vi "maxigauge_get_p.vi"(8 "err_in":errorcluster, 10 "sensor_number":i32=1, 11 "visa_in":refnum<visa-resource-name>="COM8") -> (0 "err_out":errorcluster, 2 "pressure":dbl caption="Torr", 3 "visa_out":refnum<visa-resource-name>, 4 "status":bool)   [LabVIEW 2019]
panel:
  out "read_2":string
  out "read_1":string
  out "status_ack":bool
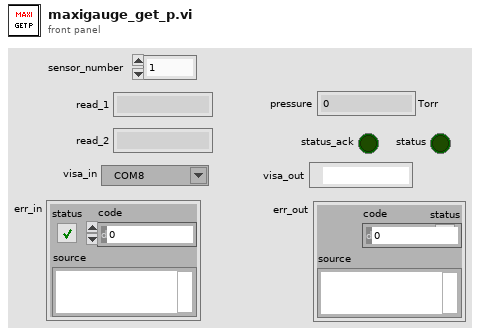
[diagram p1: front panel]
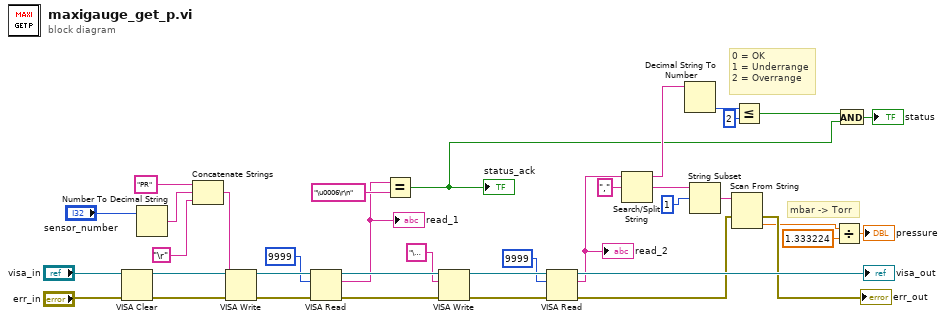
[diagram p0: block diagram]
diagram:
  # "0 = OK\n1 = Underrange\n2 = Overrange"
  # "mbar -> Torr"
  n1 = VISA Clear(VISA resource name="visa_in", error in (no error)="err_in") -> (VISA resource name out=w13:refnum<visa-resource-name>, error out=w11:errorcluster)
  n2 = Number To Decimal String(number="sensor_number") -> (decimal integer string=w16:string)  [unwired: 1 in]
  n3 = Concatenate Strings("PR" ("string"), w16, "\r") -> (w17:string)
  n4 = VISA Write(VISA resource name=w13, write buffer=w17, error in (no error)=w11) -> (VISA resource name out=w36:refnum<visa-resource-name>, error out=w37:errorcluster)  [unwired: 1 out]
  n5 = VISA Read(VISA resource name=w36, byte count=u32 9999, error in (no error)=w37) -> (VISA resource name out=w34:refnum<visa-resource-name>, read buffer=w23:string, error out=w33:errorcluster)  [unwired: 1 out]
  "read_1" <- w23
  n6 = Equal?(x=w23, y="\u0006\r\n") -> (x = y?=w20:bool)
  "status_ack" <- w20
  n7 = VISA Write(VISA resource name=w34, write buffer="\u0005", error in (no error)=w33) -> (VISA resource name out=w32:refnum<visa-resource-name>, error out=w31:errorcluster)  [unwired: 1 out]
  n8 = VISA Read(VISA resource name=w32, byte count=u32 9999, error in (no error)=w31) -> (VISA resource name out=→"visa_out":refnum<visa-resource-name>, read buffer=w29:string, error out=w7:errorcluster)  [unwired: 1 out]
  "read_2" <- w29
  n9 = Search/Split String(string=w29, search string/char (-)=",") -> (substring before match=w25:string, match + rest of string=w27:string)  [unwired: 1 in, 1 out]
  n10 = Decimal String To Number(string=w25) -> (number=w2:i32)  [unwired: 2 in, 1 out]
  n11 = String Subset(string=w27, offset (0)=1) -> (substring=w14:string)  [unwired: 1 in]
  n12 = Scan From String(input string=w14, error in=w7) -> (error out=→"err_out":errorcluster, output 1=w3:dbl)  [unwired: 3 in, 2 out]
  n13 = Less Or Equal?(x=w2, y=2) -> (x <= y?=w21:bool)
  n14 = Divide(x=w3, y=1.333224) -> (x/y=→"pressure":dbl)
  n15 = And(x=w21, y=w20) -> (x .and. y?=→"status":bool)
